vi "LabVIEW调用本地大模型.vi"() -> ()   [LabVIEW 2023, in "LabVIEW LLM.lvlib"]
uses:
  LabVIEW LLM.lvlib
  openai_message.ctl
  chat-role.ctl
  chat-completion req.ctl
  <vilib>/Utility/error.llb/Trim Whitespace One-Sided.vi
  labview-ai-share/LabVIEW AI Base.lvlib
panel:
  in  "API Key":string
  in  "system prompt":string="你是一名测试测量领域的专家。" caption="System提示词"
  in  "Stream?":bool
  in  "temperature (default: 0.8)":dbl=0.8 format="%.1f"
  in  "max tokens (default: 4096)":u32=4096
  in  "Clear":bool
  in  "model URL":string="http://localhost:1234/v1"
  in  "Send":bool
  in  "Input":string="请用通俗易懂的话解释一下奈奎斯特采样定理。"
  in  "选择本地模型":string(combo)
  out "error out":errorcluster
  in  "STOP":bool
  out "对话":string
  # "LabVIEW调用本地大模型"
  # "参数"
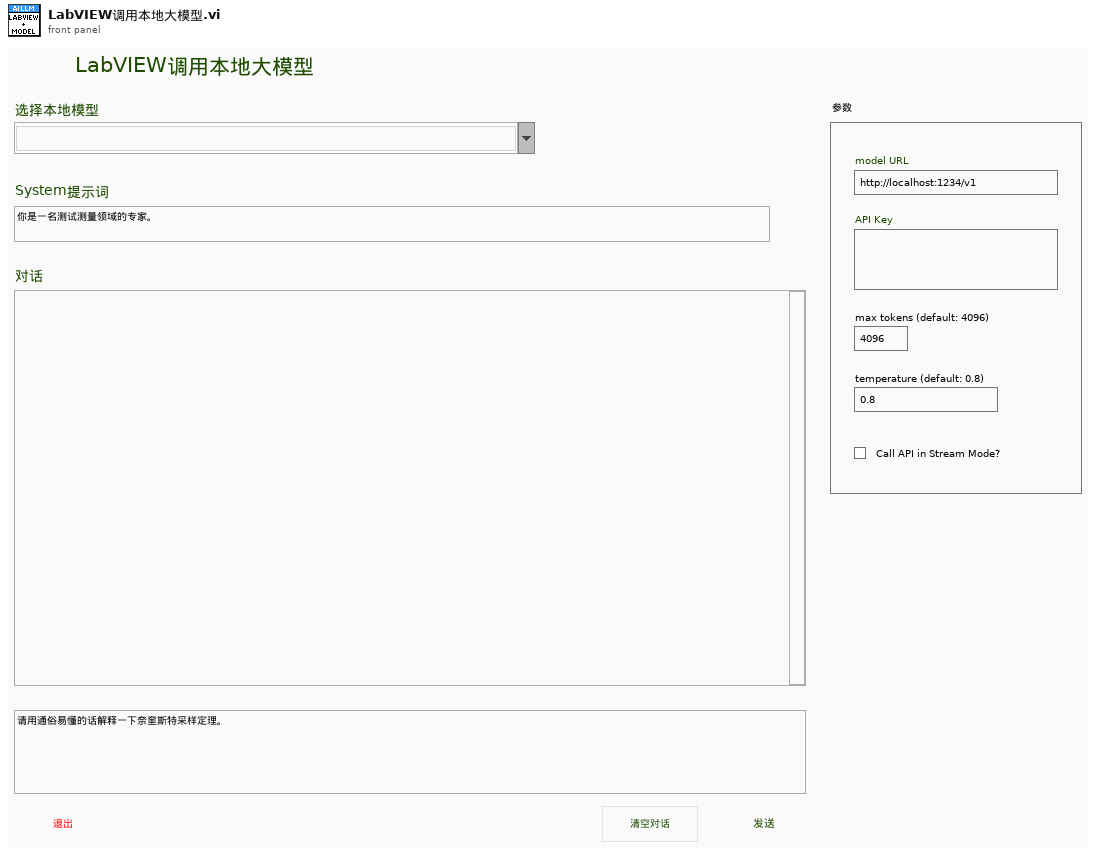
[diagram p1: front panel]
types:
  T1 = typedef "LabVIEW LLM.lvlib/openai_message.ctl" = cluster{"role":T2, "content":string, "reasoning":string}
  T2 = typedef "LabVIEW LLM.lvlib/chat-role.ctl" = enum16{"system", "user", "assistant"}
  T3 = typedef "LabVIEWHTTPClient.lvlib/ClientHandle.ctl" = refnum<k1>
  T4 = typedef "LabVIEW LLM.lvlib/chat-completion req.ctl" = cluster{"model":string, "messages":T1[], "max_tokens":u32, "temperature":dbl, "stream":bool, "reasoning":cluster{"effort":enum16{"high", "medium", "low"}, "exclude":bool}}
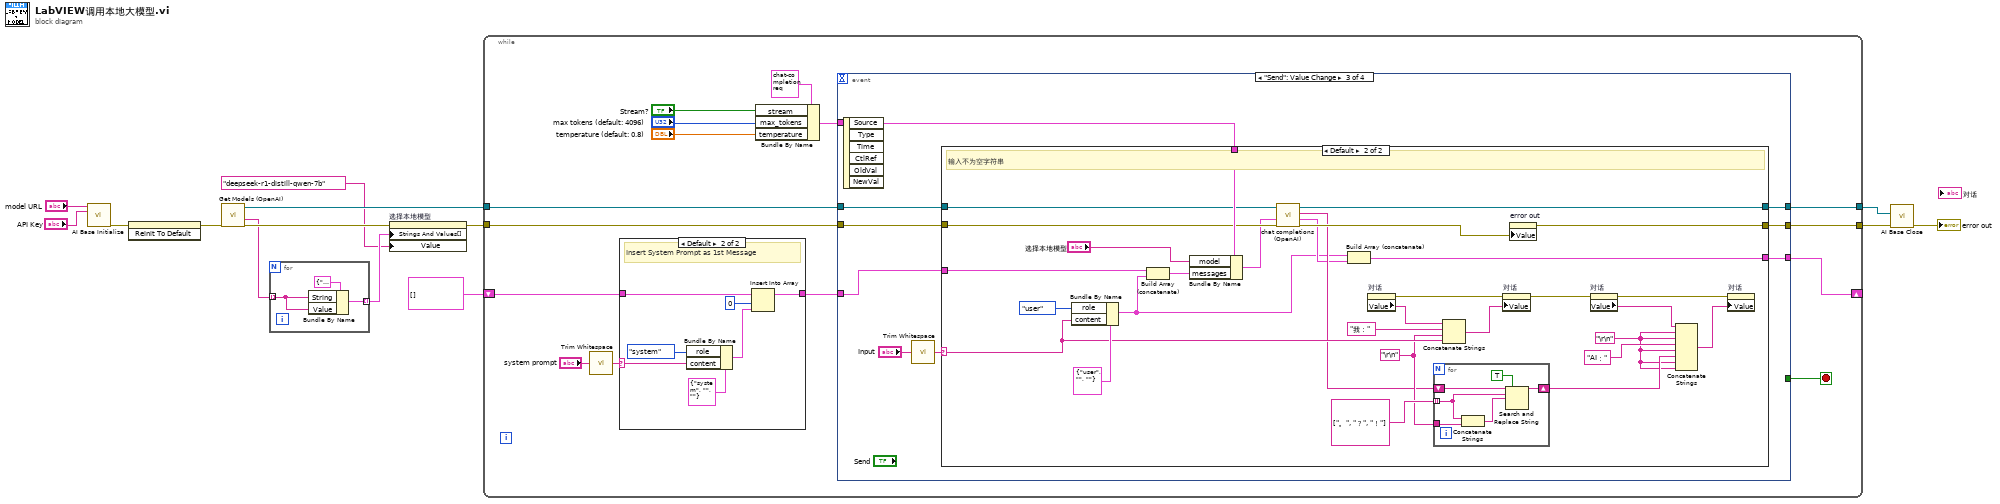
[diagram p0: block diagram]
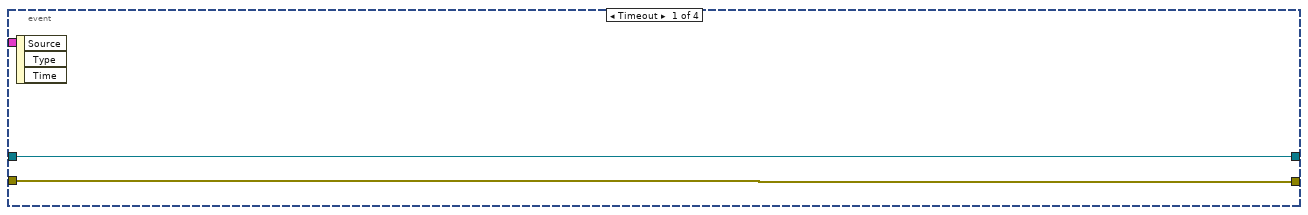
[diagram p3: hidden frame]
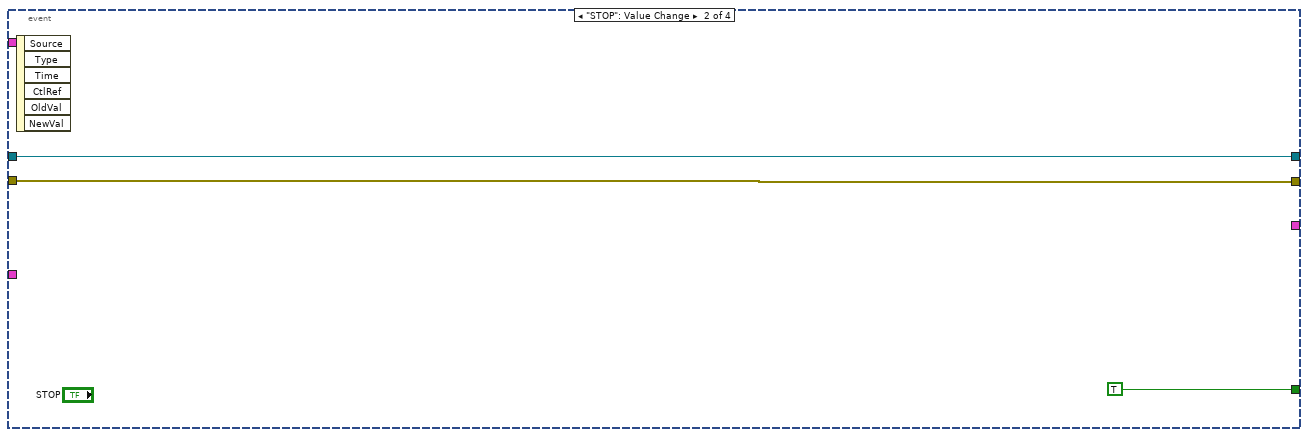
[diagram p4: hidden frame]
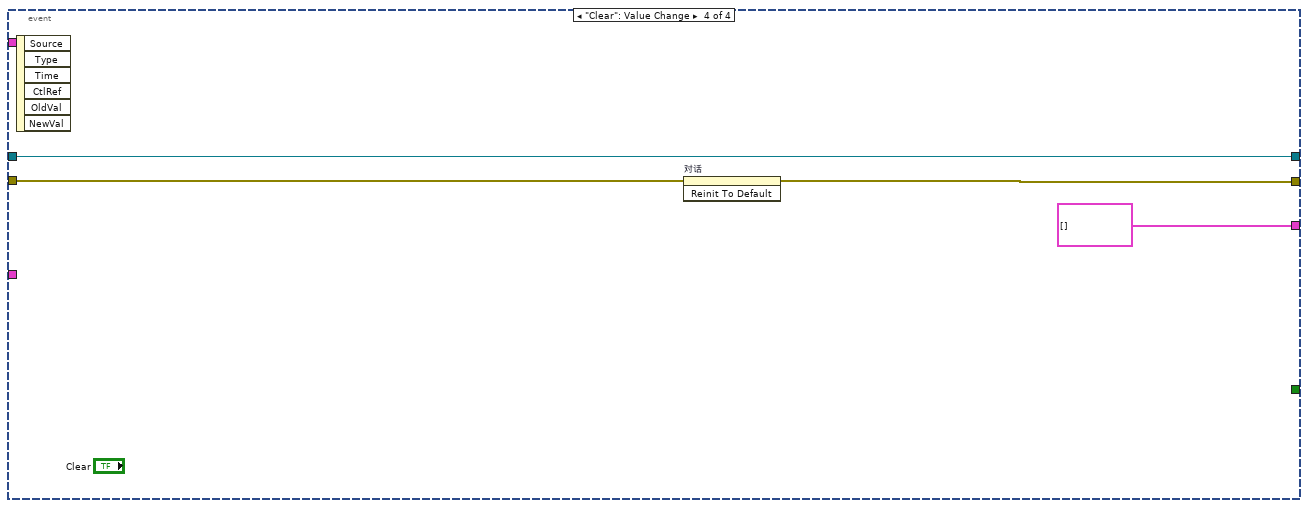
[diagram p6: hidden frame]
diagram:
  n1 = call "AI Base Initialize.vi"("OpenAI API URL"="model URL", "API Key"="API Key") -> ("error out"=w4:errorcluster)  [unwired: 11 in, 2 out]
  n2 = invoke on="Input" class="Str" method="Reinit To Default"(error in=w4) -> (error out=w6:errorcluster)  [unwired: 2 in, 2 out]
  n3 = call "Get Models (OpenAI).vi"("error in (no error)"=w6) -> ("error out"=w9:errorcluster, "Available Models"=w7:string[], "Refnum out"=w11:T3)  [unwired: 7 in, 1 out]
  n4 = for {
    tunnel: [w16] -> w10 mode=indexing
    tunnel: w7 -> [w15] mode=indexing
    n5 = Bundle By Name(cluster=cluster{"String":string, "Value":string} {"String"="", "Value"=""} ("Cluster"), "String"=w15, "Value"=w15) -> (w16:cluster{"String":string, "Value":string})
  }
  n6 = property on="选择本地模型" class="CmbBox"(error in=w9, "Strings And Values[]"=w10, "Value"="deepseek-r1-distill-qwen-7b" ("选择本地模型")) -> (error out=w8:errorcluster)  [unwired: 1 in, 1 out]
  n7 = while {
    tunnel: w11 -> [w31]
    tunnel: w8 -> [w30]
    tunnel: [w29] -> w14
    tunnel: [w28] -> w13
    shift-right: [w27] -> _
    shift-left: T1[] [] ("previous messages") -> [w21]
    stop <- w32 stop-if-true
    n8 = call <vilib>:"Trim Whitespace.vi"("string"="system prompt") -> ("trimmed string"=w18:string)  [unwired: 1 in]
    n9 = case shown="Default" w18 {
      selector: w18 -> [_ w40]
      tunnel: w21 -> [w33 w35]
      tunnel: [w33 w37] -> w20
      frame "" {
      }
      frame Default {
        # "Insert System Prompt as 1st Message"
        n10 = Bundle By Name(cluster=T1 {"role"=enum."system", "content"="", "reasoning"=""} ("message"), "role"=enum16{"system", "user", "assistant"}."system", "content"=w40) -> (w36:T1)
        n11 = Insert Into Array(array=w35, index=0, new element=w36) -> (w37:T1[])
      }
    }
    n12 = Bundle By Name(cluster=T4 {"model"="", "messages"=[{"role"=enum."user", "content"="", "reasoning"=""}], "max_tokens"=4096, "temperature"=0.7, "stream"=FALSE, "reasoning"={"effort"=enum."low", "exclude"=FALSE}}, "stream"="Stream?", "max_tokens"="max tokens (default: 4096)", "temperature"="temperature (default: 0.8)") -> (w26:T4)
    n13 = event shown="[2] \"Send\": Value Change" {
      selector: _ -> [_ _ _ _]
      dyn-events: _ -> [_ _ _ _]
      timeout: _ -> [_ _ _ _]
      tunnel: [_ TRUE _ _] -> w32
      tunnel: w31 -> [w42 w44 w51 w96]
      tunnel: w30 -> [w41 w43 w53 w95]
      tunnel: w26 -> [_ _ w54 _]
      tunnel: [w42 w44 w52 w96] -> w29
      tunnel: [w41 w43 w50 w94] -> w28
      tunnel: [_ _ w48 T1[] []] -> w27
      tunnel: w20 -> [_ _ w47 _]
      event Timeout {
        n14 = event-data() -> ()  [unwired: 1 in, 3 out]
      }
      event "STOP": Value Change {
        n15 = event-data() -> ()  [unwired: 1 in, 6 out]
      }
      event "Send": Value Change {
        n16 = event-data() -> ()  [unwired: 1 in, 6 out]
        n17 = call <vilib>:"Trim Whitespace.vi"("string"="Input") -> ("trimmed string"=w46:string)  [unwired: 1 in]
        n18 = case shown="Default" w46 {
          selector: w46 -> [_ w75]
          tunnel: w54 -> [_ w87]
          tunnel: w53 -> [w57 w86]
          tunnel: [w56 w82] -> w52
          tunnel: w51 -> [w56 w81]
          tunnel: [w57 w80] -> w50
          tunnel: [w55 w62] -> w48
          tunnel: w47 -> [w55 w60]
          frame "" {
          }
          frame Default {
            w58 = "\r\n"
            w65 = "\r\n"
            # "输入不为空字符串"
            n19 = Bundle By Name(cluster=T1 {"role"=enum."user", "content"="", "reasoning"=""} ("messages"), "role"=enum16{"system", "user", "assistant"}."user", "content"=w75) -> (w61:T1)
            n20 = Build Array (concatenate)(w60, w61) -> (w83:T1[])
            n21 = Bundle By Name(cluster=w87, "model"="选择本地模型", "messages"=w83) -> (w85:T4)
            n22 = call "chat completions (OpenAI).vi"("error in"=w86, "chat-completion req"=w85, "Refnum in"=w81) -> ("error out"=w79:errorcluster, "previous messages"=w63:T1[], "Answer content"=w64:string, "Refnum out"=w82:T3)  [unwired: 4 in, 1 out]
            n23 = Build Array (concatenate)(w61, w63) -> (w62:T1[])
            n24 = property on="对话" class="Str"() -> (error out=w78:errorcluster, "Value"=w77:string)  [unwired: 2 in, 1 out]
            n25 = for {
              tunnel: string[] ["。", "？", "！"] ("search string") -> [w91] mode=indexing
              tunnel: w65 -> [w89]
              shift-right: [w93] -> w67
              shift-left: w64 -> [w88]
              n26 = Concatenate Strings(w91, w89) -> (w90:string)
              n27 = Search and Replace String(replace all?=TRUE ("replace all? (F)"), input string=w88, search string=w91, replace string=w90) -> (result string=w93:string)  [unwired: 4 in, 3 out]
            }
            n28 = Concatenate Strings(w77, "我：" ("string"), w65, w75) -> (w76:string)
            n29 = property on="对话" class="Str"(error in=w78, "Value"=w76) -> (error out=w70:errorcluster)  [unwired: 1 in, 1 out]
            n30 = property on="error out" class="Clust (strict)"("Value"=w79) -> (error out=w80:errorcluster)  [unwired: 2 in, 1 out]
            n31 = property on="对话" class="Str"(error in=w70) -> (error out=w71:errorcluster, "Value"=w68:string)  [unwired: 1 in, 1 out]
            n32 = Concatenate Strings(w68, w58, w58, "AI：" ("string"), w58, w67, w58, w58) -> (w69:string)
            n33 = property on="对话" class="Str"(error in=w71, "Value"=w69) -> ()  [unwired: 1 in, 2 out]
          }
        }
      }
      event "Clear": Value Change {
        n34 = event-data() -> ()  [unwired: 1 in, 6 out]
        n35 = invoke on="对话" class="Str" method="Reinit To Default"(error in=w95) -> (error out=w94:errorcluster)  [unwired: 2 in, 2 out]
      }
    }
  }
  n36 = call "AI Base Close.vi"("error in"=w13, "Http Refnum in"=w14) -> ("error out"=→"error out":errorcluster)  [unwired: 9 in]
